vi "Send command return raw text.vi"(0 "VISA resource":refnum<visa-resource-name>, 1 "Action":T1, 2 "Periodic(F)":bool, 5 "d(0.0)":dbl, 7 "n(0)":i32, 11 "error in (no error)":errorcluster) -> (4 "VISA resource out":refnum<visa-resource-name>, 6 "Return Data":variant, 8 "Return string":string, 10 "Sendt string":string, 13 "Reply received":bool, 14 "Reply Expected":bool, 15 "error out":errorcluster)   [LabVIEW 2011]
doc: "Sends the actual command values, waits for the return strnig, but does not interprate it."
uses:
  PCP Commands.ctl
  emi Lib/Basic/0 - General/Time/Private/emi_Time offset holder.vi
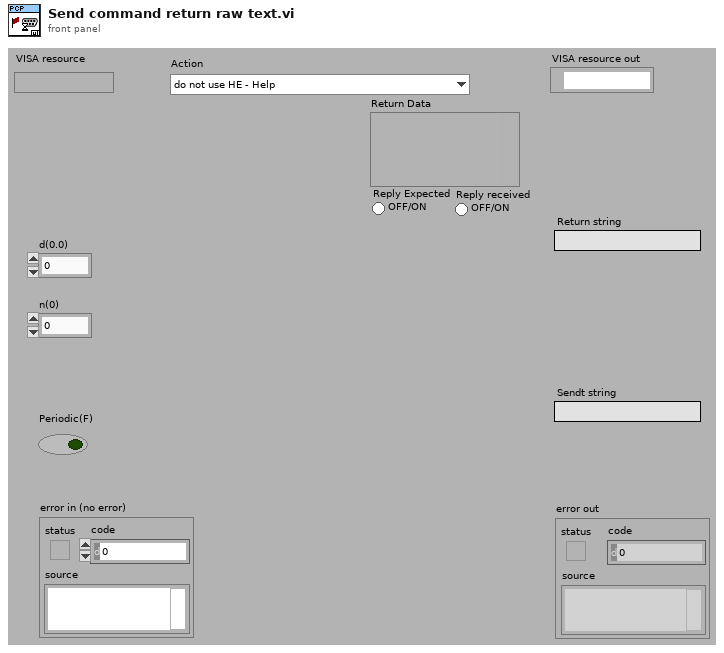
[diagram p1: front panel]
types:
  T1 = typedef "PCP Commands.ctl" = enum16{"do not use HE - Help", "RDd - Most used inputs", "RA - All analog inputs", "RE n Reset DO n", "SE n Set DO n", "RP - Get digital inputs", "VA d Set AO A  Motor Volt", "VB d Set AO B  Cable Resistance", "VEr - Get Version", "DYp - Depth counter", "DR - Reset Depth Counter", "DS n Set Depth options(0-3)", "do not use ME - Manual mode enabled", "MD - Manual mode disabled", "ID - Get ID(2001)", "TS - Get Timestamp", "TO d(s)  Set timeout", "do not use LO n Start Loop Mode(1,2)", "AL n RD&LO variation", "ST - Stop Loop Mode"}
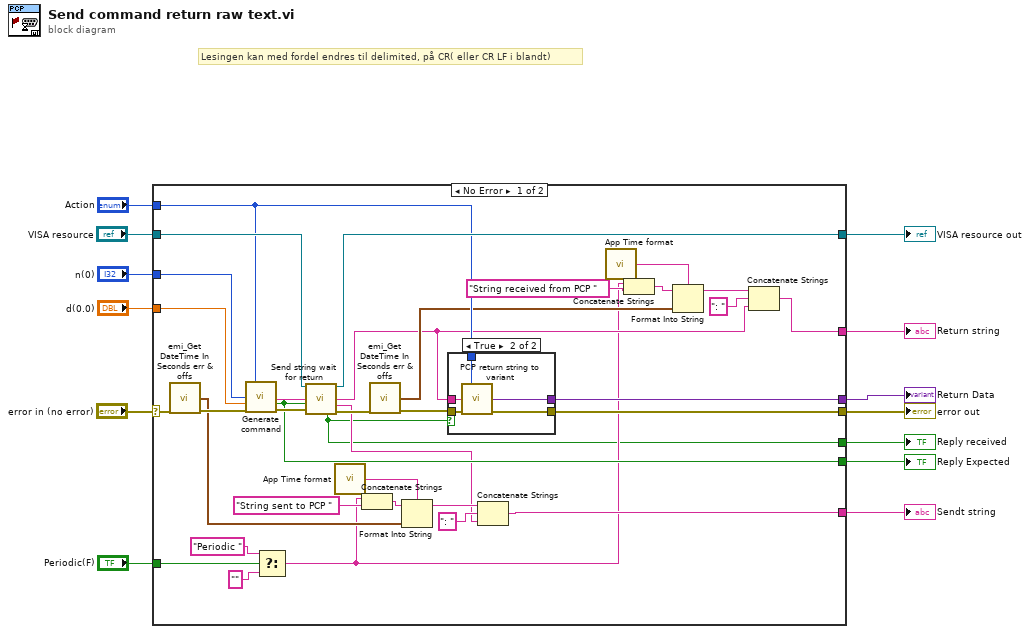
[diagram p0: block diagram]
diagram:
  # "Lesingen kan med fordel endres til delimited, på CR( eller CR LF i blandt)"
  n1 = case shown="No Error" "error in (no error)" {
    selector: "error in (no error)" -> [w38 w55]
    tunnel: [w42 w55] -> w12
    tunnel: "VISA resource" -> [w45 w56]
    tunnel: [w44 w56] -> w10
    tunnel: "Action" -> [w41 _]
    tunnel: "n(0)" -> [w47 _]
    tunnel: "d(0.0)" -> [w48 _]
    tunnel: [w21 _] -> w6
    tunnel: [w28 _] -> w5
    tunnel: [w40 _] -> w4
    tunnel: [w39 _] -> w3
    tunnel: "Periodic(F)" -> [w17 _]
    tunnel: [w14 _] -> w1
    frame No Error {
      n2 = call "emi_Get DateTime In Seconds err & offs.vi"("error in (no error)"=w38) -> ("Time"=w31:timestamp, "error out"=w37:errorcluster)  [unwired: 13 in]
      n3 = call "Generate command.vi"("Action"=w41, "n(0)"=w47, "d(0.0)"=w48, "error IO"=w37) -> ("Command string"=w43:string, "Reply expected"=w39:bool, "error out"=w46:errorcluster)  [unwired: 9 in]
      n4 = Select(t="Periodic " ("initial string"), s=w17, f="" ("initial string")) -> (s? t:f=w15:string)
      n5 = call "Send string wait for return.vi"("VISA resource"=w45, "Command string"=w43, "Reply expected"=w39, "error IO"=w46) -> ("VISA resource out"=w44:refnum<visa-resource-name>, "Reply string"=w22:string, "Transmitted"=w29:string, "Received Reply"=w14:bool, "error out"=w36:errorcluster)  [unwired: 7 in]
      n6 = call "App Time format.vi"() -> ("App timeformat"=w34:string)  [unwired: 15 in]
      n7 = Concatenate Strings(w15, "String sent to PCP " ("initial string")) -> (w20:string)
      n8 = call "emi_Get DateTime In Seconds err & offs.vi"("error in (no error)"=w36) -> ("Time"=w23:timestamp, "error out"=w35:errorcluster)  [unwired: 13 in]
      n9 = Format Into String(format string=w34, initial string=w20, w31) -> (resulting string=w32:string)  [unwired: 1 in, 1 out]
      n10 = case shown="True" w14 {
        tunnel: w35 -> [w49 w54]
        tunnel: [w49 w53] -> w42
        tunnel: w41 -> [_ w52]
        tunnel: w22 -> [_ w51]
        tunnel: [_ w50] -> w40
        frame False {
        }
        frame True {
          n11 = call "PCP return string to variant.vi"("Action"=w52, "PCP return string"=w51, "error in (no error)"=w54) -> ("Data"=w50:variant, "error out"=w53:errorcluster)  [unwired: 11 in]
        }
      }
      n12 = Concatenate Strings(w32, ": " ("string"), w29) -> (w28:string)
      n13 = call "App Time format.vi"() -> ("App timeformat"=w27:string)  [unwired: 15 in]
      n14 = Concatenate Strings(w15, "String received from PCP " ("initial string")) -> (w16:string)
      n15 = Format Into String(format string=w27, initial string=w16, w23) -> (resulting string=w25:string)  [unwired: 1 in, 1 out]
      n16 = Concatenate Strings(w25, ": " ("string"), w22) -> (w21:string)
    }
    frame Error {
    }
  }
  "error out" <- w12
  "VISA resource out" <- w10
  "Sendt string" <- w5
  "Return string" <- w6
  "Return Data" <- w4
  "Reply Expected" <- w3
  "Reply received" <- w1
